vi "read Txt Files.vi"(10 "file path (use dialog)":path) -> (1 "error out":errorcluster, 2 "number":T1)   [LabVIEW 2017] (continued)
Velocity(0.1mm0/s)¡G\t0.000000\tVoltage¡G\t0.007751\nReal Periold(ms)¡G\t1\tEncoder Position(0.1mm)¡G\t0.000000\tVelocity(0.1mm0/s)¡G\t0.000000\tVoltage¡G\t0.020477\nReal Periold(ms)¡G\t1\tEncoder Position(0.1mm)¡G\t0.000000\tVelocity(0.1mm0/s)¡G\t0.000000\tVoltage¡G\t-0.002441\nReal Periold(ms)¡G\t1\tEncoder Position(0.1mm)¡G\t0.000000\tVelocity(0.1mm0/s)¡G\t0.000000\tVoltage¡G\t-0.006897\nReal Periold(ms)¡G\t1\tEncoder Position(0.1mm)¡G\t0.000000\tVelocity(0.1mm0/s)¡G\t0.000000\tVoltage¡G\t-0.011353\nReal Periold(ms)¡G\t1\tEncoder Position(0.1mm)¡G\t0.000000\tVelocity(0.1mm0/s)¡G\t0.000000\tVoltage¡G\t-0.000854\nReal Periold(ms)¡G\t1\tEncoder Position(0.1mm)¡G\t0.000000\tVelocity(0.1mm0/s)¡G\t0.000000\tVoltage¡G\t-0.012634\nReal Periold(ms)¡G\t1\tEncoder Position(0.1mm)¡G\t0.000000\tVelocity(0.1mm0/s)¡G\t0.000000\tVoltage¡G\t0.000092\nReal Periold(ms)¡G\t1\tEncoder Position(0.1mm)¡G\t0.000000\tVelocity(0.1mm0/s)¡G\t0.000000\tVoltage¡G\t-0.014862\nReal Periold(ms)¡G\t1\tEncoder Position(0.1mm)¡G\t0.000000\tVelocity(0.1mm0/s)¡G\t0.000000\tVoltage¡G\t-0.011047\nReal Periold(ms)¡G\t1\tEncoder Position(0.1mm)¡G\t0.000000\tVelocity(0.1mm0/s)¡G\t0.000000\tVoltage¡G\t0.001068\nReal Periold(ms)¡G\t1\tEncoder Position(0.1mm)¡G\t0.000000\tVelocity(0.1mm0/s)¡G\t0.000000\tVoltage¡G\t0.006775\nReal Periold(ms)¡G\t1\tEncoder Position(0.1mm)¡G\t0.000000\tVelocity(0.1mm0/s)¡G\t0.000000\tVoltage¡G\t-0.002136\nReal Periold(ms)¡G\t1\tEncoder Position(0.1mm)¡G\t0.000000\tVelocity(0.1mm0/s)¡G\t0.000000\tVoltage¡G\t-0.004364\nReal Periold(ms)¡G\t1\tEncoder Position(0.1mm)¡G\t0.000000\tVelocity(0.1mm0/s)¡G\t0.000000\tVoltage¡G\t-0.005005\nReal Periold(ms)¡G\t1\tEncoder Position(0.1mm)¡G\t0.000000\tVelocity(0.1mm0/s)¡G\t0.000000\tVoltage¡G\t0.004547\nReal Periold(ms)¡G\t1\tEncoder Position(0.1mm)¡G\t0.000000\tVelocity(0.1mm0/s)¡G\t0.000000\tVoltage¡G\t-0.007538\nReal Periold(ms)¡G\t1\tEncoder Position(0.1mm)¡G\t0.000000\tVelocity(0.1mm0/s)¡G\t0.000000\tVoltage¡G\t-0.004669\nReal Periold(ms)¡G\t1\tEncoder Position(0.1mm)¡G\t0.000000\tVelocity(0.1mm0/s)¡G\t0.000000\tVoltage¡G\t-0.001495\nReal Periold(ms)¡G\t1\tEncoder Position(0.1mm)¡G\t0.000000\tVelocity(0.1mm0/s)¡G\t0.000000\tVoltage¡G\t-0.010406\nReal Periold(ms)¡G\t1\tEncoder Position(0.1mm)¡G\t0.000000\tVelocity(0.1mm0/s)¡G\t0.000000\tVoltage¡G\t-0.007538\nReal Periold(ms)¡G\t1\tEncoder Position(0.1mm)¡G\t0.000000\tVelocity(0.1mm0/s)¡G\t0.000000\tVoltage¡G\t0.004547\nReal Periold(ms)¡G\t1\tEncoder Position(0.1mm)¡G\t0.000000\tVelocity(0.1mm0/s)¡G\t0.000000\tVoltage¡G\t0.030334\nReal Periold(ms)¡G\t1\tEncoder Position(0.1mm)¡G\t0.000000\tVelocity(0.1mm0/s)¡G\t0.000000\tVoltage¡G\t-0.001160\nReal Periold(ms)¡G\t1\tEncoder Position(0.1mm)¡G\t0.000000\tVelocity(0.1mm0/s)¡G\t0.000000\tVoltage¡G\t-0.005615\nReal Periold(ms)¡G\t1\tEncoder Position(0.1mm)¡G\t0.000000\tVelocity(0.1mm0/s)¡G\t0.000000\tVoltage¡G\t0.007751\nReal Periold(ms)¡G\t1\tEncoder Position(0.1mm)¡G\t0.000000\tVelocity(0.1mm0/s)¡G\t0.000000\tVoltage¡G\t0.077118\nReal Periold(ms)¡G\t1\tEncoder Position(0.1mm)¡G\t0.000000\tVelocity(0.1mm0/s)¡G\t0.000000\tVoltage¡G\t0.000732\nReal Periold(ms)¡G\t1\tEncoder Position(0.1mm)¡G\t0.000000\tVelocity(0.1mm0/s)¡G\t0.000000\tVoltage¡G\t0.002319\nReal Periold(ms)¡G\t1\tEncoder Position(0.1mm)¡G\t0.000000\tVelocity(0.1mm0/s)¡G\t0.000000\tVoltage¡G\t0.007111\nReal Periold(ms)¡G\t1\tEncoder Position(0.1mm)¡G\t0.000000\tVelocity(0.1mm0/s)¡G\t0.000000\tVoltage¡G\t-0.006897\nReal Periold(ms)¡G\t1\tEncoder Position(0.1mm)¡G\t0.000000\tVelocity(0.1mm0/s)¡G\t0.000000\tVoltage¡G\t0.003296\nReal Periold(ms)¡G\t1\tEncoder Position(0.1mm)¡G\t0.000000\tVelocity(0.1mm0/s)¡G\t0.000000\tVoltage¡G\t-0.004028\nReal Periold(ms)¡G\t1\tEncoder Position(0.1mm)¡G\t0.000000\tVelocity(0.1mm0/s)¡G\t0.000000\tVoltage¡G\t0.011230\nReal Periold(ms)¡G\t1\tEncoder Position(0.1mm)¡G\t0.000000\tVelocity(0.1mm0/s)¡G\t0.000000\tVoltage¡G\t0.002655\nReal Periold(ms)¡G\t1\tEncoder Position(0.1mm)¡G\t0.000000\tVelocity(0.1mm0/s)¡G\t0.000000\tVoltage¡G\t-0.003723\nReal Periold(ms)¡G\t1\tEncoder Position(0.1mm)¡G\t0.000000\tVelocity(0.1mm0/s)¡G\t0.000000\tVoltage¡G\t-0.008484\nReal Periold(ms)¡G\t1\tEncoder Position(0.1mm)¡G\t0.000000\tVelocity(0.1mm0/s)¡G\t0.000000\tVoltage¡G\t-0.000214\nReal Periold(ms)¡G\t1\tEncoder Position(0.1mm)¡G\t0.000000\tVelocity(0.1mm0/s)¡G\t0.000000\tVoltage¡G\t-0.000214\nReal Periold(ms)¡G\t1\tEncoder Position(0.1mm)¡G\t0.000000\tVelocity(0.1mm0/s)¡G\t0.000000\tVoltage¡G\t0.007751\nReal Periold(ms)¡G\t1\tEncoder Position(0.1mm)¡G\t0.000000\tVelocity(0.1mm0/s)¡G\t0.000000\tVoltage¡G\t-0.000214\nReal Periold(ms)¡G\t1\tEncoder Position(0.1mm)¡G\t0.000000\tVelocity(0.1mm0/s)¡G\t0.000000\tVoltage¡G\t-0.006256\nReal Periold(ms)¡G\t1\tEncoder Position(0.1mm)¡G\t0.000000\tVelocity(0.1mm0/s)¡G\t0.000000\tVoltage¡G\t0.008698\nReal Periold(ms)¡G\t1\tEncoder Position(0.1mm)¡G\t0.000000\tVelocity(0.1mm0/s)¡G\t0.000000\tVoltage¡G\t-0.009766\nReal Periold(ms)¡G\t1\tEncoder Position(0.1mm)¡G\t0.000000\tVelocity(0.1mm0/s)¡G\t0.000000\tVoltage¡G\t-0.000214\nReal Periold(ms)¡G\t1\tEncoder Position(0.1mm)¡G\t0.000000\tVelocity(0.1mm0/s)¡G\t0.000000\tVoltage¡G\t-0.002777\nReal Periold(ms)¡G\t1\tEncoder Position(0.1mm)¡G\t0.000000\tVelocity(0.1mm0/s)¡G\t0.000000\tVoltage¡G\t-0.001160\nReal Periold(ms)¡G\t1\tEncoder Position(0.1mm)¡G\t0.000000\tVelocity(0.1mm0/s)¡G\t0.000000\tVoltage¡G\t-0.002136\nReal Periold(ms)¡G\t1\tEncoder Position(0.1mm)¡G\t0.000000\tVelocity(0.1mm0/s)¡G\t0.000000\tVoltage¡G\t0.006134\nReal Periold(ms)¡G\t1\tEncoder Position(0.1mm)¡G\t0.000000\tVelocity(0.1mm0/s)¡G\t0.000000\tVoltage¡G\t0.001373\nReal Periold(ms)¡G\t1\tEncoder Position(0.1mm)¡G\t0.000000\tVelocity(0.1mm0/s)¡G\t0.000000\tVoltage¡G\t0.001678\nReal Periold(ms)¡G\t1\tEncoder Position(0.1mm)¡G\t0.000000\tVelocity(0.1mm0/s)¡G\t0.000000\tVoltage¡G\t0.002319\nReal Periold(ms)¡G\t1\tEncoder Position(0.1mm)¡G\t0.000000\tVelocity(0.1mm0/s)¡G\t0.000000\tVoltage¡G\t0.002014\nReal Periold(ms)¡G\t1\tEncoder Position(0.1mm)¡G\t0.000000\tVelocity(0.1mm0/s)¡G\t0.000000\tVoltage¡G\t-0.009460\nReal Periold(ms)¡G\t1\tEncoder Position(0.1mm)¡G\t0.000000\tVelocity(0.1mm0/s)¡G\t0.000000\tVoltage¡G\t-0.002136\nReal Periold(ms)¡G\t1\tEncoder Position(0.1mm)¡G\t0.000000\tVelocity(0.1mm0/s)¡G\t0.000000\tVoltage¡G\t-0.022186\nReal Periold(ms)¡G\t1\tEncoder Position(0.1mm)¡G\t0.000000\tVelocity(0.1mm0/s)¡G\t0.000000\tVoltage¡G\t-0.008484\nReal Periold(ms)¡G\t1\tEncoder Position(0.1mm)¡G\t0.000000\tVelocity(0.1mm0/s)¡G\t0.000000\tVoltage¡G\t-0.010071\nReal Periold(ms)¡G\t1\tEncoder Position(0.1mm)¡G\t0.000000\tVelocity(0.1mm0/s)¡G\t0.000000\tVoltage¡G\t-0.009125\nReal Periold(ms)¡G\t1\tEncoder Position(0.1mm)¡G\t0.000000\tVelocity(0.1mm0/s)¡G\t0.000000\tVoltage¡G\t-0.010406\nReal Periold(ms)¡G\t1\tEncoder Position(0.1mm)¡G\t0.000000\tVelocity(0.1mm0/s)¡G\t0.000000\tVoltage¡G\t-0.008179\nReal Periold(ms)¡G\t1\tEncoder Position(0.1mm)¡G\t0.000000\tVelocity(0.1mm0/s)¡G\t0.000000\tVoltage¡G\t0.004242\nReal Periold(ms)¡G\t1\tEncoder Position(0.1mm)¡G\t0.000000\tVelocity(0.1mm0/s)¡G\t0.000000\tVoltage¡G\t-0.008484\nReal Periold(ms)¡G\t1\tEncoder Position(0.1mm)¡G\t0.000000\tVelocity(0.1mm0/s)¡G\t0.000000\tVoltage¡G\t0.009338\nReal Periold(ms)¡G\t1\tEncoder Position(0.1mm)¡G\t0.000000\tVelocity(0.1mm0/s)¡G\t0.000000\tVoltage¡G\t0.013458\nReal Periold(ms)¡G\t1\tEncoder Position(0.1mm)¡G\t0.000000\tVelocity(0.1mm0/s)¡G\t0.000000\tVoltage¡G\t0.001678\nReal Periold(ms)¡G\t1\tEncoder Position(0.1mm)¡G\t0.000000\tVelocity(0.1mm0/s)¡G\t0.000000\tVoltage¡G\t-0.001801\nReal Periold(ms)¡G\t1\tEncoder Position(0.1mm)¡G\t0.000000\tVelocity(0.1mm0/s)¡G\t0.000000\tVoltage¡G\t-0.002777\nReal Periold(ms)¡G\t1\tEncoder Position(0.1mm)¡G\t0.000000\tVelocity(0.1mm0/s)¡G\t0.000000\tVoltage¡G\t-0.002777\nReal Periold(ms)¡G\t1\tEncoder Position(0.1mm)¡G\t0.000000\tVelocity(0.1mm0/s)¡G\t0.000000\tVoltage¡G\t-0.012939\nReal Periold(ms)¡G\t1\tEncoder Position(0.1mm)¡G\t0.000000\tVelocity(0.1mm0/s)¡G\t0.000000\tVoltage¡G\t-0.006897\nReal Periold(ms)¡G\t1\tEncoder Position(0.1mm)¡G\t0.000000\tVelocity(0.1mm0/s)¡G\t0.000000\tVoltage¡G\t0.002655\nReal Periold(ms)¡G\t1\tEncoder Position(0.1mm)¡G\t0.000000\tVelocity(0.1mm0/s)¡G\t0.000000\tVoltage¡G\t0.001678\nReal Periold(ms)¡G\t1\tEncoder Position(0.1mm)¡G\t0.000000\tVelocity(0.1mm0/s)¡G\t0.000000\tVoltage¡G\t-0.005615\nReal Periold(ms)¡G\t1\tEncoder Position(0.1mm)¡G\t0.000000\tVelocity(0.1mm0/s)¡G\t0.000000\tVoltage¡G\t-0.007538\nReal Periold(ms)¡G\t1\tEncoder Position(0.1mm)¡G\t0.000000\tVelocity(0.1mm0/s)¡G\t0.000000\tVoltage¡G\t-0.001495\nReal Periold(ms)¡G\t1\tEncoder Position(0.1mm)¡G\t0.000000\tVelocity(0.1mm0/s)¡G\t0.000000\tVoltage¡G\t0.006470\nReal Periold(ms)¡G\t1\tEncoder Position(0.1mm)¡G\t0.000000\tVelocity(0.1mm0/s)¡G\t0.000000\tVoltage¡G\t-0.001495\nReal Periold(ms)¡G\t1\tEncoder Position(0.1mm)¡G\t0.000000\tVelocity(0.1mm0/s)¡G\t0.000000\tVoltage¡G\t-0.012634\nReal Periold(ms)¡G\t1\tEncoder Position(0.1mm)¡G\t0.000000\tVelocity(0.1mm0/s)¡G\t0.000000\tVoltage¡G\t-0.009125\nReal Periold(ms)¡G\t1\tEncoder Position(0.1mm)¡G\t0.000000\tVelocity(0.1mm0/s)¡G\t0.000000\tVoltage¡G\t-0.002441\nReal Periold(ms)¡G\t1\tEncoder Position(0.1mm)¡G\t0.000000\tVelocity(0.1mm0/s)¡G\t0.000000\tVoltage¡G\t0.006775\nReal Periold(ms)¡G\t1\tEncoder Position(0.1mm)¡G\t0.000000\tVelocity(0.1mm0/s)¡G\t0.000000\tVoltage¡G\t0.009644\nReal Periold(ms)¡G\t1\tEncoder Position(0.1mm)¡G\t0.000000\tVelocity(0.1mm0/s)¡G\t0.000000\tVoltage¡G\t-0.004669\nReal Periold(ms)¡G\t1\tEncoder Position(0.1mm)¡G\t0.000000\tVelocity(0.1mm0/s)¡G\t0.000000\tVoltage¡G\t-0.014862\nReal Periold(ms)¡G\t1\tEncoder Position(0.1mm)¡G\t0.000000\tVelocity(0.1mm0/s)¡G\t0.000000\tVoltage¡G\t0.004547\nReal Periold(ms)¡G\t1\tEncoder Position(0.1mm)¡G\t0.000000\tVelocity(0.1mm0/s)¡G\t0.000000\tVoltage¡G\t0.005524\nReal Periold(ms)¡G\t1\tEncoder Position(0.1mm)¡G\t0.000000\tVelocity(0.1mm0/s)¡G\t0.000000\tVoltage¡G\t-0.012634\nReal Periold(ms)¡G\t1\tEncoder Position(0.1mm)¡G\t0.000000\tVelocity(0.1mm0/s)¡G\t0.000000\tVoltage¡G\t0.006470\nReal Periold(ms)¡G\t1\tEncoder Position(0.1mm)¡G\t0.000000\tVelocity(0.1mm0/s)¡G\t0.000000\tVoltage¡G\t-0.008179\nReal Periold(ms)¡G\t1\tEncoder Position(0.1mm)¡G\t0.000000\tVelocity(0.1mm0/s)¡G\t0.000000\tVoltage¡G\t-0.001160\nReal Periold(ms)¡G\t1\tEncoder Position(0.1mm)¡G\t0.000000\tVelocity(0.1mm0/s)¡G\t0.000000\tVoltage¡G\t0.016663\nReal Periold(ms)¡G\t1\tEncoder Position(0.1mm)¡G\t0.000000\tVelocity(0.1mm0/s)¡G\t0.000000\tVoltage¡G\t0.006775\nReal Periold(ms)¡G\t1\tEncoder Position(0.1mm)¡G\t0.000000\tVelocity(0.1mm0/s)¡G\t0.000000\tVoltage¡G\t0.006134\nReal Periold(ms)¡G\t1\tEncoder Position(0.1mm)¡G\t0.000000\tVelocity(0.1mm0/s)¡G\t0.000000\tVoltage¡G\t-0.009460\nReal Periold(ms)¡G\t1\tEncoder Position(0.1mm)¡G\t0.000000\tVelocity(0.1mm0/s)¡G\t0.000000\tVoltage¡G\t-0.009460\nReal Periold(ms)¡G\t1\tEncoder Position(0.1mm)¡G\t0.000000\tVelocity(0.1mm0/s)¡G\t0.000000\tVoltage¡G\t-0.016144\nReal Periold(ms)¡G\t1\tEncoder Position(0.1mm)¡G\t0.000000\tVelocity(0.1mm0/s)¡G\t0.000000\tVoltage¡G\t-0.005615\nReal Periold(ms)¡G\t1\tEncoder Position(0.1mm)¡G\t0.000000\tVelocity(0.1mm0/s)¡G\t0.000000\tVoltage¡G\t-0.003387\nReal Periold(ms)¡G\t1\tEncoder Position(0.1mm)¡G\t0.000000\tVelocity(0.1mm0/s)¡G\t0.000000\tVoltage¡G\t0.030029\nReal Periold(ms)¡G\t1\tEncoder Position(0.1mm)¡G\t0.000000\tVelocity(0.1mm0/s)¡G\t0.000000\tVoltage¡G\t-0.001801\nReal Periold(ms)¡G\t1\tEncoder Position(0.1mm)¡G\t0.000000\tVelocity(0.1mm0/s)¡G\t0.000000\tVoltage¡G\t-0.012939\nReal Periold(ms)¡G\t1\tEncoder Position(0.1mm)¡G\t0.000000\tVelocity(0.1mm0/s)¡G\t0.000000\tVoltage¡G\t-0.004364\nReal Periold(ms)¡G\t1\tEncoder Position(0.1mm)¡G\t0.000000\tVelocity(0.1mm0/s)¡G\t0.000000\tVoltage¡G\t-0.003387\nReal Periold(ms)¡G\t1\tEncoder Position(0.1mm)¡G\t0.000000\tVelocity(0.1mm0/s)¡G\t0.000000\tVoltage¡G\t-0.002777\nReal Periold(ms)¡G\t1\tEncoder Position(0.1mm)¡G\t0.000000\tVelocity(0.1mm0/s)¡G\t0.000000\tVoltage¡G\t0.005188\nReal Periold(ms)¡G\t1\tEncoder Position(0.1mm)¡G\t0.000000\tVelocity(0.1mm0/s)¡G\t0.000000\tVoltage¡G\t-0.003387\nReal Periold(ms)¡G\t1\tEncoder Position(0.1mm)¡G\t0.000000\tVelocity(0.1mm0/s)¡G\t0.000000\tVoltage¡G\t-0.007233\nReal Periold(ms)¡G\t1\tEncoder Position(0.1mm)¡G\t0.000000\tVelocity(0.1mm0/s)¡G\t0.000000\tVoltage¡G\t-0.004364\nReal Periold(ms)¡G\t1\tEncoder Position(0.1mm)¡G\t0.000000\tVelocity(0.1mm0/s)¡G\t0.000000\tVoltage¡G\t0.002960\nReal Periold(ms)¡G\t1\tEncoder Position(0.1mm)¡G\t0.000000\tVelocity(0.1mm0/s)¡G\t0.000000\tVoltage¡G\t-0.007843\nReal Periold(ms)¡G\t1\tEncoder Position(0.1mm)¡G\t0.000000\tVelocity(0.1mm0/s)¡G\t0.000000\tVoltage¡G\t0.008057\nReal Periold(ms)¡G\t1\tEncoder Position(0.1mm)¡G\t0.000000\tVelocity(0.1mm0/s)¡G\t0.000000\tVoltage¡G\t-0.004364\nReal Periold(ms)¡G\t1\tEncoder Position(0.1mm)¡G\t0.000000\tVelocity(0.1mm0/s)¡G\t0.000000\tVoltage¡G\t-0.000854\nReal Periold(ms)¡G\t1\tEncoder Position(0.1mm)¡G\t0.000000\tVelocity(0.1mm0/s)¡G\t0.000000\tVoltage¡G\t0.002319\nReal Periold(ms)¡G\t1\tEncoder Position(0.1mm)¡G\t0.000000\tVelocity(0.1mm0/s)¡G\t0.000000\tVoltage¡G\t0.003601\nReal Periold(ms)¡G\t1\tEncoder Position(0.1mm)¡G\t0.000000\tVelocity(0.1mm0/s)¡G\t0.000000\tVoltage¡G\t0.019501\nReal Periold(ms)¡G\t1\tEncoder Position(0.1mm)¡G\t0.000000\tVelocity(0.1mm0/s)¡G\t0.000000\tVoltage¡G\t0.014740\nReal Periold(ms)¡G\t1\tEncoder Position(0.1mm)¡G\t0.000000\tVelocity(0.1mm0/s)¡G\t0.000000\tVoltage¡G\t0.003906\nReal Periold(ms)¡G\t1\tEncoder Position(0.1mm)¡G\t0.000000\tVelocity(0.1mm0/s)¡G\t0.000000\tVoltage¡G\t-0.002136\nReal Periold(ms)¡G\t1\tEncoder Position(0.1mm)¡G\t0.000000\tVelocity(0.1mm0/s)¡G\t0.000000\tVoltage¡G\t0.000427\nReal Periold(ms)¡G\t1\tEncoder Position(0.1mm)¡G\t0.000000\tVelocity(0.1mm0/s)¡G\t0.000000\tVoltage¡G\t-0.006897\nReal Periold(ms)¡G\t1\tEncoder Position(0.1mm)¡G\t0.000000\tVelocity(0.1mm0/s)¡G\t0.000000\tVoltage¡G\t-0.006897\nReal Periold(ms)¡G\t1\tEncoder Position(0.1mm)¡G\t0.000000\tVelocity(0.1mm0/s)¡G\t0.000000\tVoltage¡G\t-0.003387\nReal Periold(ms)¡G\t1\tEncoder Position(0.1mm)¡G\t0.000000\tVelocity(0.1mm0/s)¡G\t0.000000\tVoltage¡G\t0.004242\nReal Periold(ms)¡G\t1\tEncoder Position(0.1mm)¡G\t0.000000\tVelocity(0.1mm0/s)¡G\t0.000000\tVoltage¡G\t-0.000854\nReal Periold(ms)¡G\t1\tEncoder Position(0.1mm)¡G\t0.000000\tVelocity(0.1mm0/s)¡G\t0.000000\tVoltage¡G\t-0.002441\nReal Periold(ms)¡G\t1\tEncoder Position(0.1mm)¡G\t0.000000\tVelocity(0.1mm0/s)¡G\t0.000000\tVoltage¡G\t-0.000549\nReal Periold(ms)¡G\t1\tEncoder Position(0.1mm)¡G\t0.000000\tVelocity(0.1mm0/s)¡G\t0.000000\tVoltage¡G\t0.004547\nReal Periold(ms)¡G\t1\tEncoder Position(0.1mm)¡G\t0.000000\tVelocity(0.1mm0/s)¡G\t0.000000\tVoltage¡G\t-0.006256\nReal Periold(ms)¡G\t1\tEncoder Position(0.1mm)¡G\t0.000000\tVelocity(0.1mm0/s)¡G\t0.000000\tVoltage¡G\t0.009338\nReal Periold(ms)¡G\t1\tEncoder Position(0.1mm)¡G\t0.000000\tVelocity(0.1mm0/s)¡G\t0.000000\tVoltage¡G\t-0.008820\nReal Periold(ms)¡G\t1\tEncoder Position(0.1mm)¡G\t0.000000\tVelocity(0.1mm0/s)¡G\t0.000000\tVoltage¡G\t0.006470\nReal Periold(ms)¡G\t1\tEncoder Position(0.1mm)¡G\t0.000000\tVelocity(0.1mm0/s)¡G\t0.000000\tVoltage¡G\t-0.002777\nReal Periold(ms)¡G\t1\tEncoder Position(0.1mm)¡G\t0.000000\tVelocity(0.1mm0/s)¡G\t0.000000\tVoltage¡G\t0.044037\nReal Periold(ms)¡G\t1\tEncoder Position(0.1mm)¡G\t0.000000\tVelocity(0.1mm0/s)¡G\t0.000000\tVoltage¡G\t-0.004364\nReal Periold(ms)¡G\t1\tEncoder Position(0.1mm)¡G\t0.000000\tVelocity(0.1mm0/s)¡G\t0.000000\tVoltage¡G\t-0.002441\nReal Periold(ms)¡G\t1\tEncoder Position(0.1mm)¡G\t0.000000\tVelocity(0.1mm0/s)¡G\t0.000000\tVoltage¡G\t-0.005310\nReal Periold(ms)¡G\t1\tEncoder Position(0.1mm)¡G\t0.000000\tVelocity(0.1mm0/s)¡G\t0.000000\tVoltage¡G\t-0.005005\nReal Periold(ms)¡G\t1\tEncoder Position(0.1mm)¡G\t0.000000\tVelocity(0.1mm0/s)¡G\t0.000000\tVoltage¡G\t-0.002136\nReal Periold(ms)¡G\t1\tEncoder Position(0.1mm)¡G\t0.000000\tVelocity(0.1mm0/s)¡G\t0.000000\tVoltage¡G\t0.004242\nReal Periold(ms)¡G\t1\tEncoder Position(0.1mm)¡G\t0.000000\tVelocity(0.1mm0/s)¡G\t0.000000\tVoltage¡G\t0.005829\nReal Periold(ms)¡G\t1\tEncoder Position(0.1mm)¡G\t0.000000\tVelocity(0.1mm0/s)¡G\t0.000000\tVoltage¡G\t-0.003387\nReal Periold(ms)¡G\t1\tEncoder Position(0.1mm)¡G\t0.000000\tVelocity(0.1mm0/s)¡G\t0.000000\tVoltage¡G\t0.005524\nReal Periold(ms)¡G\t1\tEncoder Position(0.1mm)¡G\t0.000000\tVelocity(0.1mm0/s)¡G\t0.000000\tVoltage¡G\t0.000427\nReal Periold(ms)¡G\t1\tEncoder Position(0.1mm)¡G\t0.000000\tVelocity(0.1mm0/s)¡G\t0.000000\tVoltage¡G\t0.006775\nReal Periold(ms)¡G\t1\tEncoder Position(0.1mm)¡G\t0.000000\tVelocity(0.1mm0/s)¡G\t0.000000\tVoltage¡G\t0.005524\nReal Periold(ms)¡G\t1\tEncoder Position(0.1mm)¡G\t0.000000\tVelocity(0.1mm0/s)¡G\t0.000000\tVoltage¡G\t-0.014862\nReal Periold(ms)¡G\t1\tEncoder Position(0.1mm)¡G\t0.000000\tVelocity(0.1mm0/s)¡G\t0.000000\tVoltage¡G\t-0.007233\nReal Periold(ms)¡G\t1\tEncoder Position(0.1mm)¡G\t0.000000\tVelocity(0.1mm0/s)¡G\t0.000000\tVoltage¡G\t-0.009125\nReal Periold(ms)¡G\t1\tEncoder Position(0.1mm)¡G\t0.000000\tVelocity(0.1mm0/s)¡G\t0.000000\tVoltage¡G\t0.001678\nReal Periold(ms)¡G\t1\tEncoder Position(0.1mm)¡G\t0.000000\tVelocity(0.1mm0/s)¡G\t0.000000\tVoltage¡G\t0.007416\nReal Periold(ms)¡G\t1\tEncoder Position(0.1mm)¡G\t0.000000\tVelocity(0.1mm0/s)¡G\t0.000000\tVoltage¡G\t-0.006592\nReal Periold(ms)¡G\t1\tEncoder Position(0.1mm)¡G\t0.000000\tVelocity(0.1mm0/s)¡G\t0.000000\tVoltage¡G\t-0.004669\nReal Periold(ms)¡G\t1\tEncoder Position(0.1mm)¡G\t0.000000\tVelocity(0.1mm0/s)¡G\t0.000000\tVoltage¡G\t-0.015167\nReal Periold(ms)¡G\t1\tEncoder Position(0.1mm)¡G\t0.000000\tVelocity(0.1mm0/s)¡G\t0.000000\tVoltage¡G\t0.002014\nReal Periold(ms)¡G\t1\tEncoder Position(0.1mm)¡G\t0.000000\tVelocity(0.1mm0/s)¡G\t0.000000\tVoltage¡G\t0.021759\nReal Periold(ms)¡G\t1\tEncoder Position(0.1mm)¡G\t0.000000\tVelocity(0.1mm0/s)¡G\t0.000000\tVoltage¡G\t0.018250\nReal Periold(ms)¡G\t1\tEncoder Position(0.1mm)¡G\t0.000000\tVelocity(0.1mm0/s)¡G\t0.000000\tVoltage¡G\t-0.005951\nReal Periold(ms)¡G\t1\tEncoder Position(0.1mm)¡G\t0.000000\tVelocity(0.1mm0/s)¡G\t0.000000\tVoltage¡G\t-0.010406\nReal Periold(ms)¡G\t1\tEncoder Position(0.1mm)¡G\t0.000000\tVelocity(0.1mm0/s)¡G\t0.000000\tVoltage¡G\t-0.009125\nReal Periold(ms)¡G\t1\tEncoder Position(0.1mm)¡G\t0.000000\tVelocity(0.1mm0/s)¡G\t0.000000\tVoltage¡G\t-0.006256\nReal Periold(ms)¡G\t1\tEncoder Position(0.1mm)¡G\t0.000000\tVelocity(0.1mm0/s)¡G\t0.000000\tVoltage¡G\t-0.018372\nReal Periold(ms)¡G\t1\tEncoder Position(0.1mm)¡G\t0.000000\tVelocity(0.1mm0/s)¡G\t0.000000\tVoltage¡G\t0.002655\nReal Periold(ms)¡G\t1\tEncoder Position(0.1mm)¡G\t0.000000\tVelocity(0.1mm0/s)¡G\t0.000000\tVoltage¡G\t-0.007233\nReal Periold(ms)¡G\t1\tEncoder Position(0.1mm)¡G\t0.000000\tVelocity(0.1mm0/s)¡G\t0.000000\tVoltage¡G\t-0.003723\nReal Periold(ms)¡G\t1\tEncoder Position(0.1mm)¡G\t0.000000\tVelocity(0.1mm0/s)¡G\t0.000000\tVoltage¡G\t-0.006256\nReal Periold(ms)¡G\t1\tEncoder Position(0.1mm)¡G\t0.000000\tVelocity(0.1mm0/s)¡G\t0.000000\tVoltage¡G\t0.000732\nReal Periold(ms)¡G\t1\tEncoder Position(0.1mm)¡G\t0.000000\tVelocity(0.1mm0/s)¡G\t0.000000\tVoltage¡G\t-0.011047\nReal Periold(ms)¡G\t1\tEncoder Position(0.1mm)¡G\t0.000000\tVelocity(0.1mm0/s)¡G\t0.000000\tVoltage¡G\t-0.018982\nReal Periold(ms)¡G\t1\tEncoder Position(0.1mm)¡G\t0.000000\tVelocity(0.1mm0/s)¡G\t0.000000\tVoltage¡G\t-0.023132\nReal Periold(ms)¡G\t1\tEncoder Position(0.1mm)¡G\t0.000000\tVelocity(0.1mm0/s)¡G\t0.000000\tVoltage¡G\t-0.011047\nReal Periold(ms)¡G\t1\tEncoder Position(0.1mm)¡G\t0.000000\tVelocity(0.1mm0/s)¡G\t0.000000\tVoltage¡G\t0.002319\nReal Periold(ms)¡G\t1\tEncoder Position(0.1mm)¡G\t0.000000\tVelocity(0.1mm0/s)¡G\t0.000000\tVoltage¡G\t-0.000214\nReal Periold(ms)¡G\t1\tEncoder Position(0.1mm)¡G\t0.000000\tVelocity(0.1mm0/s)¡G\t0.000000\tVoltage¡G\t-0.014862\nReal Periold(ms)¡G\t1\tEncoder Position(0.1mm)¡G\t0.000000\tVelocity(0.1mm0/s)¡G\t0.000000\tVoltage¡G\t0.008698\nReal Periold(ms)¡G\t1\tEncoder Position(0.1mm)¡G\t0.000000\tVelocity(0.1mm0/s)¡G\t0.000000\tVoltage¡G\t0.013153\nReal Periold(ms)¡G\t1\tEncoder Position(0.1mm)¡G\t0.000000\tVelocity(0.1mm0/s)¡G\t0.000000\tVoltage¡G\t-0.007233\nReal Periold(ms)¡G\t1\tEncoder Position(0.1mm)¡G\t0.000000\tVelocity(0.1mm0/s)¡G\t0.000000\tVoltage¡G\t-0.005310\nReal Periold(ms)¡G\t1\tEncoder Position(0.1mm)¡G\t0.000000\tVelocity(0.1mm0/s)¡G\t0.000000\tVoltage¡G\t0.003296\nReal Periold(ms)¡G\t1\tEncoder Position(0.1mm)¡G\t0.000000\tVelocity(0.1mm0/s)¡G\t0.000000\tVoltage¡G\t-0.002136\nReal Periold(ms)¡G\t1\tEncoder Position(0.1mm)¡G\t0.000000\tVelocity(0.1mm0/s)¡G\t0.000000\tVoltage¡G\t0.008698\nReal Periold(ms)¡G\t1\tEncoder Position(0.1mm)¡G\t0.000000\tVelocity(0.1mm0/s)¡G\t0.000000\tVoltage¡G\t0.003296\nReal Periold(ms)¡G\t1\tEncoder Position(0.1mm)¡G\t0.000000\tVelocity(0.1mm0/s)¡G\t0.000000\tVoltage¡G\t0.001678\nReal Periold(ms)¡G\t1\tEncoder Position(0.1mm)¡G\t0.000000\tVelocity(0.1mm0/s)¡G\t0.000000\tVoltage¡G\t-0.004028\nReal Periold(ms)¡G\t1\tEncoder Position(0.1mm)¡G\t0.000000\tVelocity(0.1mm0/s)¡G\t0.000000\tVoltage¡G\t0.006134\nReal Periold(ms)¡G\t1\tEncoder Position(0.1mm)¡G\t0.000000\tVelocity(0.1mm0/s)¡G\t0.000000\tVoltage¡G\t-0.002136\nReal Periold(ms)¡G\t1\tEncoder Position(0.1mm)¡G\t0.000000\tVelocity(0.1mm0/s)¡G\t0.000000\tVoltage¡G\t-0.009460\nReal Periold(ms)¡G\t1\tEncoder Position(0.1mm)¡G\t0.000000\tVelocity(0.1mm0/s)¡G\t0.000000\tVoltage¡G\t0.000732\nReal Periold(ms)¡G\t1\tEncoder Position(0.1mm)¡G\t0.000000\tVelocity(0.1mm0/s)¡G\t0.000000\tVoltage¡G\t-0.011993\nReal Periold(ms)¡G\t1\tEncoder Position(0.1mm)¡G\t0.000000\tVelocity(0.1mm0/s)¡G\t0.000000\tVoltage¡G\t-0.016449\nReal Periold(ms)¡G\t1\tEncoder Position(0.1mm)¡G\t0.000000\tVelocity(0.1mm0/s)¡G\t0.000000\tVoltage¡G\t0.010925\nReal Periold(ms)¡G\t1\tEncoder Position(0.1mm)¡G\t0.000000\tVelocity(0.1mm0/s)¡G\t0.000000\tVoltage¡G\t0.014099\nReal Periold(ms)¡G\t1\tEncoder Position(0.1mm)¡G\t0.000000\tVelocity(0.1mm0/s)¡G\t0.000000\tVoltage¡G\t0.060883\nReal Periold(ms)¡G\t1\tEncoder Position(0.1mm)¡G\t0.000000\tVelocity(0.1mm0/s)¡G\t0.000000\tVoltage¡G\t0.004242\nReal Periold(ms)¡G\t1\tEncoder Position(0.1mm)¡G\t0.000000\tVelocity(0.1mm0/s)¡G\t0.000000\tVoltage¡G\t0.000732\nReal Periold(ms)¡G\t1\tEncoder Position(0.1mm)¡G\t0.000000\tVelocity(0.1mm0/s)¡G\t0.000000\tVoltage¡G\t-0.001495\nReal Periold(ms)¡G\t1\tEncoder Position(0.1mm)¡G\t0.000000\tVelocity(0.1mm0/s)¡G\t0.000000\tVoltage¡G\t-0.009460\nReal Periold(ms)¡G\t1\tEncoder Position(0.1mm)¡G\t0.000000\tVelocity(0.1mm0/s)¡G\t0.000000\tVoltage¡G\t-0.008820\nReal Periold(ms)¡G\t1\tEncoder Position(0.1mm)¡G\t0.000000\tVelocity(0.1mm0/s)¡G\t0.000000\tVoltage¡G\t-0.001495\nReal Periold(ms)¡G\t1\tEncoder Position(0.1mm)¡G\t0.000000\tVelocity(0.1mm0/s)¡G\t0.000000\tVoltage¡G\t0.006775\nReal Periold(ms)¡G\t1\tEncoder Position(0.1mm)¡G\t0.000000\tVelocity(0.1mm0/s)¡G\t0.000000\tVoltage¡G\t-0.005615\nReal Periold(ms)¡G\t1\tEncoder Position(0.1mm)¡G\t0.000000\tVelocity(0.1mm0/s)¡G\t0.000000\tVoltage¡G\t-0.150146\nReal Periold(ms)¡G\t1\tEncoder Position(0.1mm)¡G\t0.000000\tVelocity(0.1mm0/s)¡G\t0.000000\tVoltage¡G\t-0.001495\nReal Periold(ms)¡G\t1\tEncoder Position(0.1mm)¡G\t0.000000\tVelocity(0.1mm0/s)¡G\t0.000000\tVoltage¡G\t0.003906\nReal Periold(ms)¡G\t1\tEncoder Position(0.1mm)¡G\t0.000000\tVelocity(0.1mm0/s)¡G\t0.000000\tVoltage¡G\t-0.000214\nReal Periold(ms)¡G\t1\tEncoder Position(0.1mm)¡G\t0.000000\tVelocity(0.1mm0/s)¡G\t0.000000\tVoltage¡G\t0.009003\nReal Periold(ms)¡G\t1\tEncoder Position(0.1mm)¡G\t0.000000\tVelocity(0.1mm0/s)¡G\t0.000000\tVoltage¡G\t-0.022827\nReal Periold(ms)¡G\t1\tEncoder Position(0.1mm)¡G\t0.000000\tVelocity(0.1mm0/s)¡G\t0.000000\tVoltage¡G\t-0.002441\nReal Periold(ms)¡G\t1\tEncoder Position(0.1mm)¡G\t0.000000\tVelocity(0.1mm0/s)¡G\t0.000000\tVoltage¡G\t-0.008820\nReal Periold(ms)¡G\t1\tEncoder Position(0.1mm)¡G\t0.000000\tVelocity(0.1mm0/s)¡G\t0.000000\tVoltage¡G\t0.006470\nReal Periold(ms)¡G\t1\tEncoder Position(0.1mm)¡G\t0.000000\tVelocity(0.1mm0/s)¡G\t0.000000\tVoltage¡G\t0.023987\nReal Periold(ms)¡G\t1\tEncoder Position(0.1mm)¡G\t0.000000\tVelocity(0.1mm0/s)¡G\t0.000000\tVoltage¡G\t0.002014\nReal Periold(ms)¡G\t1\tEncoder Position(0.1mm)¡G\t0.000000\tVelocity(0.1mm0/s)¡G\t0.000000\tVoltage¡G\t-0.013275\nReal Periold(ms)¡G\t1\tEncoder Position(0.1mm)¡G\t0.000000\tVelocity(0.1mm0/s)¡G\t0.000000\tVoltage¡G\t-0.005005\nReal Periold(ms)¡G\t1\tEncoder Position(0.1mm)¡G\t0.000000\tVelocity(0.1mm0/s)¡G\t0.000000\tVoltage¡G\t-0.001801\nReal Periold(ms)¡G\t1\tEncoder Position(0.1mm)¡G\t0.000000\tVelocity(0.1mm0/s)¡G\t0.000000\tVoltage¡G\t0.004242\nReal Periold(ms)¡G\t1\tEncoder Position(0.1mm)¡G\t0.000000\tVelocity(0.1mm0/s)¡G\t0.000000\tVoltage¡G\t0.009979\nReal Periold(ms)¡G\t1\tEncoder Position(0.1mm)¡G\t0.000000\tVelocity(0.1mm0/s)¡G\t0.000000\tVoltage¡G\t0.093994\nReal Periold(ms)¡G\t1\tEncoder Position(0.1mm)¡G\t0.000000\tVelocity(0.1mm0/s)¡G\t0.000000\tVoltage¡G\t-0.006897\nReal Periold(ms)¡G\t1\tEncoder Position(0.1mm)¡G\t0.000000\tVelocity(0.1mm0/s)¡G\t0.000000\tVoltage¡G\t0.001373\nReal Periold(ms)¡G\t1\tEncoder Position(0.1mm)¡G\t0.000000\tVelocity(0.1mm0/s)¡G\t0.000000\tVoltage¡G\t0.004242\nReal Periold(ms)¡G\t1\tEncoder Position(0.1mm)¡G\t0.000000\tVelocity(0.1mm0/s)¡G\t0.000000\tVoltage¡G\t-0.005951\nReal Periold(ms)¡G\t1\tEncoder Position(0.1mm)¡G\t0.000000\tVelocity(0.1mm0/s)¡G\t0.000000\tVoltage¡G\t0.007416\nReal Periold(ms)¡G\t1\tEncoder Position(0.1mm)¡G\t0.000000\tVelocity(0.1mm0/s)¡G\t0.000000\tVoltage¡G\t0.002014\nReal Periold(ms)¡G\t1\tEncoder Position(0.1mm)¡G\t0.000000\tVelocity(0.1mm0/s)¡G\t0.000000\tVoltage¡G\t-0.008179\nReal Periold(ms)¡G\t1\tEncoder Position(0.1mm)¡G\t0.000000\tVelocity(0.1mm0/s)¡G\t0.000000\tVoltage¡G\t0.001068\nReal Periold(ms)¡G\t1\tEncoder Position(0.1mm)¡G\t0.000000\tVelocity(0.1mm0/s)¡G\t0.000000\tVoltage¡G\t0.002319\nReal Periold(ms)¡G\t1\tEncoder Position(0.1mm)¡G\t0.000000\tVelocity(0.1mm0/s)¡G\t0.000000\tVoltage¡G\t-0.008179\nReal Periold(ms)¡G\t1\tEncoder Position(0.1mm)¡G\t0.000000\tVelocity(0.1mm0/s)¡G\t0.000000\tVoltage¡G\t0.010284\nReal Periold(ms)¡G\t1\tEncoder Position(0.1mm)¡G\t0.000000\tVelocity(0.1mm0/s)¡G\t0.000000\tVoltage¡G\t0.005188\nReal Periold(ms)¡G\t1\tEncoder Position(0.1mm)¡G\t0.000000\tVelocity(0.1mm0/s)¡G\t0.000000\tVoltage¡G\t-0.000854\nReal Periold(ms)¡G\t1\tEncoder Position(0.1mm)¡G\t0.000000\tVelocity(0.1mm0/s)¡G\t0.000000\tVoltage¡G\t0.014099\nReal Periold(ms)¡G\t1\tEncoder Position(0.1mm)¡G\t0.000000\tVelocity(0.1mm0/s)¡G\t0.000000\tVoltage¡G\t-0.009766\nReal Periold(ms)¡G\t1\tEncoder Position(0.1mm)¡G\t0.000000\tVelocity(0.1mm0/s)¡G\t0.000000\tVoltage¡G\t0.000092\nReal Periold(ms)¡G\t1\tEncoder Position(0.1mm)¡G\t0.000000\tVelocity(0.1mm0/s)¡G\t0.000000\tVoltage¡G\t-0.005615\nReal Periold(ms)¡G\t1\tEncoder Position(0.1mm)¡G\t0.000000\tVelocity(0.1mm0/s)¡G\t0.000000\tVoltage¡G\t-0.005310\nReal Periold(ms)¡G\t1\tEncoder Position(0.1mm)¡G\t0.000000\tVelocity(0.1mm0/s)¡G\t0.000000\tVoltage¡G\t0.009338\nReal Periold(ms)¡G\t1\tEncoder Position(0.1mm)¡G\t0.000000\tVelocity(0.1mm0/s)¡G\t0.000000\tVoltage¡G\t0.035736\nReal Periold(ms)¡G\t1\tEncoder Position(0.1mm)¡G\t0.000000\tVelocity(0.1mm0/s)¡G\t0.000000\tVoltage¡G\t0.035736\nReal Periold(ms)¡G\t1\tEncoder Position(0.1mm)¡G\t0.000000\tVelocity(0.1mm0/s)¡G\t0.000000\tVoltage¡G\t0.052948\nReal Periold(ms)¡G\t1\tEncoder Position(0.1mm)¡G\t0.000000\tVelocity(0.1mm0/s)¡G\t0.000000\tVoltage¡G\t-0.001160\nReal Periold(ms)¡G\t1\tEncoder Position(0.1mm)¡G\t0.000000\tVelocity(0.1mm0/s)¡G\t0.000000\tVoltage¡G\t-0.001495\nReal Periold(ms)¡G\t1\tEncoder Position(0.1mm)¡G\t0.000000\tVelocity(0.1mm0/s)¡G\t0.000000\tVoltage¡G\t-0.006256\nReal Periold(ms)¡G\t1\tEncoder Position(0.1mm)¡G\t0.000000\tVelocity(0.1mm0/s)¡G\t0.000000\tVoltage¡G\t-0.043823\nReal Periold(ms)¡G\t1\tEncoder Position(0.1mm)¡G\t0.000000\tVelocity(0.1mm0/s)¡G\t0.000000\tVoltage¡G\t0.011230\nReal Periold(ms)¡G\t1\tEncoder Position(0.1mm)¡G\t0.000000\tVelocity(0.1mm0/s)¡G\t0.000000\tVoltage¡G\t-0.007233\nReal Periold(ms)¡G\t1\tEncoder Position(0.1mm)¡G\t0.000000\tVelocity(0.1mm0/s)¡G\t0.000000\tVoltage¡G\t0.030029\nReal Periold(ms)¡G\t1\tEncoder Position(0.1mm)¡G\t0.000000\tVelocity(0.1mm0/s)¡G\t0.000000\tVoltage¡G\t0.105469\nReal Periold(ms)¡G\t1\tEncoder Position(0.1mm)¡G\t0.000000\tVelocity(0.1mm0/s)¡G\t0.000000\tVoltage¡G\t-0.031097\nReal Periold(ms)¡G\t1\tEncoder Position(0.1mm)¡G\t0.000000\tVelocity(0.1mm0/s)¡G\t0.000000\tVoltage¡G\t0.001373\nReal Periold(ms)¡G\t1\tEncoder Position(0.1mm)¡G\t0.000000\tVelocity(0.1mm0/s)¡G\t0.000000\tVoltage¡G\t-0.068024\nReal Periold(ms)¡G\t1\tEncoder Position(0.1mm)¡G\t0.000000\tVelocity(0.1mm0/s)¡G\t0.000000\tVoltage¡G\t0.072998\nReal Periold(ms)¡G\t1\tEncoder Position(0.1mm)¡G\t0.000000\tVelocity(0.1mm0/s)¡G\t0.000000\tVoltage¡G\t0.008362\nReal Periold(ms)¡G\t1\tEncoder Position(0.1mm)¡G\t0.000000\tVelocity(0.1mm0/s)¡G\t0.000000\tVoltage¡G\t-0.005615\nReal Periold(ms)¡G\t1\tEncoder Position(0.1mm)¡G\t0.000000\tVelocity(0.1mm0/s)¡G\t0.000000\tVoltage¡G\t0.012512\nReal Periold(ms)¡G\t1\tEncoder Position(0.1mm)¡G\t0.000000\tVelocity(0.1mm0/s)¡G\t0.000000\tVoltage¡G\t-0.009125\nReal Periold(ms)¡G\t1\tEncoder Position(0.1mm)¡G\t0.000000\tVelocity(0.1mm0/s)¡G\t0.000000\tVoltage¡G\t0.039886\nReal Periold(ms)¡G\t1\tEncoder Position(0.1mm)¡G\t0.000000\tVelocity(0.1mm0/s)¡G\t0.000000\tVoltage¡G\t-0.004028\nReal Periold(ms)¡G\t1\tEncoder Position(0.1mm)¡G\t0.000000\tVelocity(0.1mm0/s)¡G\t0.000000\tVoltage¡G\t-0.006256\nReal Periold(ms)¡G\t1\tEncoder Position(0.1mm)¡G\t0.000000\tVelocity(0.1mm0/s)¡G\t0.000000\tVoltage¡G\t0.015381\nReal Periold(ms)¡G\t1\tEncoder Position(0.1mm)¡G\t0.000000\tVelocity(0.1mm0/s)¡G\t0.000000\tVoltage¡G\t0.009003\nReal Periold(ms)¡G\t1\tEncoder Position(0.1mm)¡G\t0.000000\tVelocity(0.1mm0/s)¡G\t0.000000\tVoltage¡G\t-0.005005\nReal Periold(ms)¡G\t1\tEncoder Position(0.1mm)¡G\t0.000000\tVelocity(0.1mm0/s)¡G\t0.000000\tVoltage¡G\t0.001068\nReal Periold(ms)¡G\t1\tEncoder Position(0.1mm)¡G\t0.000000\tVelocity(0.1mm0/s)¡G\t0.000000\tVoltage¡G\t0.067566\nReal Periold(ms)¡G\t1\tEncoder Position(0.1mm)¡G\t0.000000\tVelocity(0.1mm0/s)¡G\t0.000000\tVoltage¡G\t0.087952\nReal Periold(ms)¡G\t1\tEncoder Position(0.1mm)¡G\t0.000000\tVelocity(0.1mm0/s)¡G\t0.000000\tVoltage¡G\t0.119141\nReal Periold(ms)¡G\t1\tEncoder Position(0.1mm)¡G\t0.000000\tVelocity(0.1mm0/s)¡G\t0.000000\tVoltage¡G\t0.047852\nReal Periold(ms)¡G\t1\tEncoder Position(0.1mm)¡G\t0.000000\tVelocity(0.1mm0/s)¡G\t0.000000\tVoltage¡G\t-0.003723\nReal Periold(ms)¡G\t1\tEncoder Position(0.1mm)¡G\t0.000000\tVelocity(0.1mm0/s)¡G\t0.000000\tVoltage¡G\t-0.003387\nReal Periold(ms)¡G\t1\tEncoder Position(0.1mm)¡G\t0.000000\tVelocity(0.1mm0/s)¡G\t0.000000\tVoltage¡G\t0.000092\nReal Periold(ms)¡G\t1\tEncoder Position(0.1mm)¡G\t0.000000\tVelocity(0.1mm0/s)¡G\t0.000000\tVoltage¡G\t-0.000549\nReal Periold(ms)¡G\t1\tEncoder Position(0.1mm)¡G\t0.000000\tVelocity(0.1mm0/s)¡G\t0.000000\tVoltage¡G\t0.001068\nReal Periold(ms)¡G\t1\tEncoder Position(0.1mm)¡G\t0.000000\tVelocity(0.1mm0/s)¡G\t0.000000\tVoltage¡G\t0.005829\nReal Periold(ms)¡G\t1\tEncoder Position(0.1mm)¡G\t0.000000\tVelocity(0.1mm0/s)¡G\t0.000000\tVoltage¡G\t0.005524\nReal Periold(ms)¡G\t1\tEncoder Position(0.1mm)¡G\t0.000000\tVelocity(0.1mm0/s)¡G\t0.000000\tVoltage¡G\t-0.014862\nReal Periold(ms)¡G\t1\tEncoder Position(0.1mm)¡G\t0.000000\tVelocity(0.1mm0/s)¡G\t0.000000\tVoltage¡G\t0.010284\nReal Periold(ms)¡G\t1\tEncoder Position(0.1mm)¡G\t0.000000\tVelocity(0.1mm0/s)¡G\t0.000000\tVoltage¡G\t0.013153\nReal Periold(ms)¡G\t1\tEncoder Position(0.1mm)¡G\t0.000000\tVelocity(0.1mm0/s)¡G\t0.000000\tVoltage¡G\t-0.004364\nReal Periold(ms)¡G\t1\tEncoder Position(0.1mm)¡G\t0.000000\tVelocity(0.1mm0/s)¡G\t0.000000\tVoltage¡G\t0.020782\nReal Periold(ms)¡G\t1\tEncoder Position(0.1mm)¡G\t0.000000\tVelocity(0.1mm0/s)¡G\t0.000000\tVoltage¡G\t-0.006256\nReal Periold(ms)¡G\t1\tEncoder Position(0.1mm)¡G\t0.000000\tVelocity(0.1mm0/s)¡G\t0.000000\tVoltage¡G\t0.001678\nReal Periold(ms)¡G\t1\tEncoder Position(0.1mm)¡G\t0.000000\tVelocity(0.1mm0/s)¡G\t0.000000\tVoltage¡G\t0.015045\nReal Periold(ms)¡G\t1\tEncoder Position(0.1mm)¡G\t0.000000\tVelocity(0.1mm0/s)¡G\t0.000000\tVoltage¡G\t-0.017731\nReal Periold(ms)¡G\t1\tEncoder Position(0.1mm)¡G\t0.000000\tVelocity(0.1mm0/s)¡G\t0.000000\tVoltage¡G\t-0.015503\nReal Periold(ms)¡G\t1\tEncoder Position(0.1mm)¡G\t0.000000\tVelocity(0.1mm0/s)¡G\t0.000000\tVoltage¡G\t-0.005310\nReal Periold(ms)¡G\t1\tEncoder Position(0.1mm)¡G\t0.000000\tVelocity(0.1mm0/s)¡G\t0.000000\tVoltage¡G\t-0.002136\nReal Periold(ms)¡G\t1\tEncoder Position(0.1mm)¡G\t0.000000\tVelocity(0.1mm0/s)¡G\t0.000000\tVoltage¡G\t-0.011993\nReal Periold(ms)¡G\t1\tEncoder Position(0.1mm)¡G\t0.000000\tVelocity(0.1mm0/s)¡G\t0.000000\tVoltage¡G\t-0.003082\nReal Periold(ms)¡G\t1\tEncoder Position(0.1mm)¡G\t0.000000\tVelocity(0.1mm0/s)¡G\t0.000000\tVoltage¡G\t-0.005005\nReal Periold(ms)¡G\t1\tEncoder Position(0.1mm)¡G\t0.000000\tVelocity(0.1mm0/s)¡G\t0.000000\tVoltage¡G\t0.050079\nReal Periold(ms)¡G\t1\tEncoder Position(0.1mm)¡G\t0.000000\tVelocity(0.1mm0/s)¡G\t0.000000\tVoltage¡G\t0.012207\nReal Periold(ms)¡G\t1\tEncoder Position(0.1mm)¡G\t0.000000\tVelocity(0.1mm0/s)¡G\t0.000000\tVoltage¡G\t0.001678\nReal Periold(ms)¡G\t1\tEncoder Position(0.1mm)¡G\t0.000000\tVelocity(0.1mm0/s)¡G\t0.000000\tVoltage¡G\t-0.001160\nReal Periold(ms)¡G\t1\tEncoder Position(0.1mm)¡G\t0.000000\tVelocity(0.1mm0/s)¡G\t0.000000\tVoltage¡G\t-0.000854\nReal Periold(ms)¡G\t1\tEncoder Position(0.1mm)¡G\t0.000000\tVelocity(0.1mm0/s)¡G\t0.000000\tVoltage¡G\t-0.001801\nReal Periold(ms)¡G\t1\tEncoder Position(0.1mm)¡G\t0.000000\tVelocity(0.1mm0/s)¡G\t0.000000\tVoltage¡G\t0.002014\nReal Periold(ms)¡G\t1\tEncoder Position(0.1mm)¡G\t0.000000\tVelocity(0.1mm0/s)¡G\t0.000000\tVoltage¡G\t-0.003723\nReal Periold(ms)¡G\t1\tEncoder Position(0.1mm)¡G\t0.000000\tVelocity(0.1mm0/s)¡G\t0.000000\tVoltage¡G\t-0.013916\nReal Periold(ms)¡G\t1\tEncoder Position(0.1mm)¡G\t0.000000\tVelocity(0.1mm0/s)¡G\t0.000000\tVoltage¡G\t-0.008484\nReal Periold(ms)¡G\t1\tEncoder Position(0.1mm)¡G\t0.000000\tVelocity(0.1mm0/s)¡G\t0.000000\tVoltage¡G\t-0.013916\nReal Periold(ms)¡G\t1\tEncoder Position(0.1mm)¡G\t0.000000\tVelocity(0.1mm0/s)¡G\t0.000000\tVoltage¡G\t0.003296\nReal Periold(ms)¡G\t1\tEncoder Position(0.1mm)¡G\t0.000000\tVelocity(0.1mm0/s)¡G\t0.000000\tVoltage¡G\t0.004547\nReal Periold(ms)¡G\t1\tEncoder Position(0.1mm)¡G\t0.000000\tVelocity(0.1mm0/s)¡G\t0.000000\tVoltage¡G\t-0.002441\nReal Periold(ms)¡G\t1\tEncoder Position(0.1mm)¡G\t0.000000\tVelocity(0.1mm0/s)¡G\t0.000000\tVoltage¡G\t-0.001495\nReal Periold(ms)¡G\t1\tEncoder Position(0.1mm)¡G\t0.000000\tVelocity(0.1mm0/s)¡G\t0.000000\tVoltage¡G\t-0.015808\nReal Periold(ms)¡G\t1\tEncoder Position(0.1mm)¡G\t0.000000\tVelocity(0.1mm0/s)¡G\t0.000000\tVoltage¡G\t-0.001495\nReal Periold(ms)¡G\t1\tEncoder Position(0.1mm)¡G\t0.000000\tVelocity(0.1mm0/s)¡G\t0.000000\tVoltage¡G\t0.001678\nReal Periold(ms)¡G\t1\tEncoder Position(0.1mm)¡G\t0.000000\tVelocity(0.1mm0/s)¡G\t0.000000\tVoltage¡G\t-0.002136\nReal Periold(ms)¡G\t1\tEncoder Position(0.1mm)¡G\t0.000000\tVelocity(0.1mm0/s)¡G\t0.000000\tVoltage¡G\t-0.000214\nReal Periold(ms)¡G\t1\tEncoder Position(0.1mm)¡G\t0.000000\tVelocity(0.1mm0/s)¡G\t0.000000\tVoltage¡G\t0.007111\nReal Periold(ms)¡G\t1\tEncoder Position(0.1mm)¡G\t0.000000\tVelocity(0.1mm0/s)¡G\t0.000000\tVoltage¡G\t0.002014\nReal Periold(ms)¡G\t1\tEncoder Position(0.1mm)¡G\t0.000000\tVelocity(0.1mm0/s)¡G\t0.000000\tVoltage¡G\t-0.001495\nReal Periold(ms)¡G\t1\tEncoder Position(0.1mm)¡G\t0.000000\tVelocity(0.1mm0/s)¡G\t0.000000\tVoltage¡G\t-0.011993\nReal Periold(ms)¡G\t1\tEncoder Position(0.1mm)¡G\t0.000000\tVelocity(0.1mm0/s)¡G\t0.000000\tVoltage¡G\t-0.002777\nReal Periold(ms)¡G\t1\tEncoder Position(0.1mm)¡G\t0.000000\tVelocity(0.1mm0/s)¡G\t0.000000\tVoltage¡G\t-0.006256\nReal Periold(ms)¡G\t1\tEncoder Position(0.1mm)¡G\t0.000000\tVelocity(0.1mm0/s)¡G\t0.000000\tVoltage¡G\t-0.002777\nReal Periold(ms)¡G\t1\tEncoder Position(0.1mm)¡G\t0.000000\tVelocity(0.1mm0/s)¡G\t0.000000\tVoltage¡G\t0.001373\nReal Periold(ms)¡G\t1\tEncoder Position(0.1mm)¡G\t0.000000\tVelocity(0.1mm0/s)¡G\t0.000000\tVoltage¡G\t-0.005310\nReal Periold(ms)¡G\t1\tEncoder Position(0.1mm)¡G\t0.000000\tVelocity(0.1mm0/s)¡G\t0.000000\tVoltage¡G\t-0.003387\nReal Periold(ms)¡G\t1\tEncoder Position(0.1mm)¡G\t0.000000\tVelocity(0.1mm0/s)¡G\t0.000000\tVoltage¡G\t-0.007233\nReal Periold(ms)¡G\t1\tEncoder Position(0.1mm)¡G\t0.000000\tVelocity(0.1mm0/s)¡G\t0.000000\tVoltage¡G\t0.002960\nReal Periold(ms)¡G\t1\tEncoder Position(0.1mm)¡G\t0.000000\tVelocity(0.1mm0/s)¡G\t0.000000\tVoltage¡G\t0.000427\nReal Periold(ms)¡G\t1\tEncoder Position(0.1mm)¡G\t0.000000\tVelocity(0.1mm0/s)¡G\t0.000000\tVoltage¡G\t0.000427\nReal Periold(ms)¡G\t1\tEncoder Position(0.1mm)¡G\t0.000000\tVelocity(0.1mm0/s)¡G\t0.000000\tVoltage¡G\t-0.000549\nReal Periold(ms)¡G\t1\tEncoder Position(0.1mm)¡G\t0.000000\tVelocity(0.1mm0/s)¡G\t0.000000\tVoltage¡G\t-0.001160\nReal Periold(ms)¡G\t1\tEncoder Position(0.1mm)¡G\t0.000000\tVelocity(0.1mm0/s)¡G\t0.000000\tVoltage¡G\t-0.001801\nReal Periold(ms)¡G\t1\tEncoder Position(0.1mm)¡G\t0.000000\tVelocity(0.1mm0/s)¡G\t0.000000\tVoltage¡G\t-0.006256\nReal Periold(ms)¡G\t1\tEncoder Position(0.1mm)¡G\t0.000000\tVelocity(0.1mm0/s)¡G\t0.000000\tVoltage¡G\t0.001373\nReal Periold(ms)¡G\t1\tEncoder Position(0.1mm)¡G\t0.000000\tVelocity(0.1mm0/s)¡G\t0.000000\tVoltage¡G\t0.014435\nReal Periold(ms)¡G\t1\tEncoder Position(0.1mm)¡G\t0.000000\tVelocity(0.1mm0/s)¡G\t0.000000\tVoltage¡G\t0.005829\nReal Periold(ms)¡G\t1\tEncoder Position(0.1mm)¡G\t0.000000\tVelocity(0.1mm0/s)¡G\t0.000000\tVoltage¡G\t0.006134\nReal Periold(ms)¡G\t1\tEncoder Position(0.1mm)¡G\t0.000000\tVelocity(0.1mm0/s)¡G\t0.000000\tVoltage¡G\t0.005829\nReal Periold(ms)¡G\t1\tEncoder Position(0.1mm)¡G\t0.000000\tVelocity(0.1mm0/s)¡G\t0.000000\tVoltage¡G\t0.010590\nReal Periold(ms)¡G\t1\tEncoder Position(0.1mm)¡G\t0.000000\tVelocity(0.1mm0/s)¡G\t0.000000\tVoltage¡G\t-0.002777\nReal Periold(ms)¡G\t1\tEncoder Position(0.1mm)¡G\t0.000000\tVelocity(0.1mm0/s)¡G\t0.000000\tVoltage¡G\t0.002319\nReal Periold(ms)¡G\t1\tEncoder Position(0.1mm)¡G\t0.000000\tVelocity(0.1mm0/s)¡G\t0.000000\tVoltage¡G\t-0.000214\nReal Periold(ms)¡G\t1\tEncoder Position(0.1mm)¡G\t0.000000\tVelocity(0.1mm0/s)¡G\t0.000000\tVoltage¡G\t-0.005615\nReal Periold(ms)¡G\t1\tEncoder Position(0.1mm)¡G\t0.000000\tVelocity(0.1mm0/s)¡G\t0.000000\tVoltage¡G\t-0.018677\nReal Periold(ms)¡G\t1\tEncoder Position(0.1mm)¡G\t0.000000\tVelocity(0.1mm0/s)¡G\t0.000000\tVoltage¡G\t0.003296\nReal Periold(ms)¡G\t1\tEncoder Position(0.1mm)¡G\t0.000000\tVelocity(0.1mm0/s)¡G\t0.000000\tVoltage¡G\t0.002014\nReal Periold(ms)¡G\t1\tEncoder Position(0.1mm)¡G\t0.000000\tVelocity(0.1mm0/s)¡G\t0.000000\tVoltage¡G\t0.002960\nReal Periold(ms)¡G\t1\tEncoder Position(0.1mm)¡G\t0.000000\tVelocity(0.1mm0/s)¡G\t0.000000\tVoltage¡G\t0.001373\nReal Periold(ms)¡G\t1\tEncoder Position(0.1mm)¡G\t0.000000\tVelocity(0.1mm0/s)¡G\t0.000000\tVoltage¡G\t0.002655\nReal Periold(ms)¡G\t1\tEncoder Position(0.1mm)¡G\t0.000000\tVelocity(0.1mm0/s)¡G\t0.000000\tVoltage¡G\t0.004883\nReal Periold(ms)¡G\t1\tEncoder Position(0.1mm)¡G\t0.000000\tVelocity(0.1mm0/s)¡G\t0.000000\tVoltage¡G\t0.025238\nReal Periold(ms)¡G\t1\tEncoder Position(0.1mm)¡G\t0.000000\tVelocity(0.1mm0/s)¡G\t0.000000\tVoltage¡G\t0.009979\nReal Periold(ms)¡G\t1\tEncoder Position(0.1mm)¡G\t0.000000\tVelocity(0.1mm0/s)¡G\t0.000000\tVoltage¡G\t0.024292\nReal Periold(ms)¡G\t1\tEncoder Position(0.1mm)¡G\t0.000000\tVelocity(0.1mm0/s)¡G\t0.000000\tVoltage¡G\t0.001678\nReal Periold(ms)¡G\t1\tEncoder Position(0.1mm)¡G\t0.000000\tVelocity(0.1mm0/s)¡G\t0.000000\tVoltage¡G\t0.001678\nReal Periold(ms)¡G\t1\tEncoder Position(0.1mm)¡G\t0.000000\tVelocity(0.1mm0/s)¡G\t0.000000\tVoltage¡G\t0.000732\nReal Periold(ms)¡G\t1\tEncoder Position(0.1mm)¡G\t0.000000\tVelocity(0.1mm0/s)¡G\t0.000000\tVoltage¡G\t0.013794\nReal Periold(ms)¡G\t1\tEncoder Position(0.1mm)¡G\t0.000000\tVelocity(0.1mm0/s)¡G\t0.000000\t
